vi "Score Display - Show Web Image (LV).vi"(10 "body":string, 11 "Picture in":refnum<vi>) -> ()   [LabVIEW 2013]
uses:
  <vilib>/picture/picture.llb/imagedata.ctl
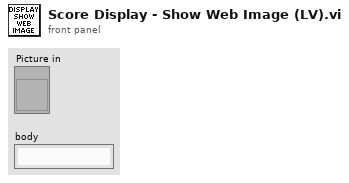
[diagram p1: front panel]
types:
  T1 = typedef "imagedata.ctl" = cluster{"image type":i32, "image depth":i32, "image":u8[], "mask":u8[], "colors":u32[], "Rectangle":cluster{"left":i16, "top":i16, "right":i16, "bottom":i16}}
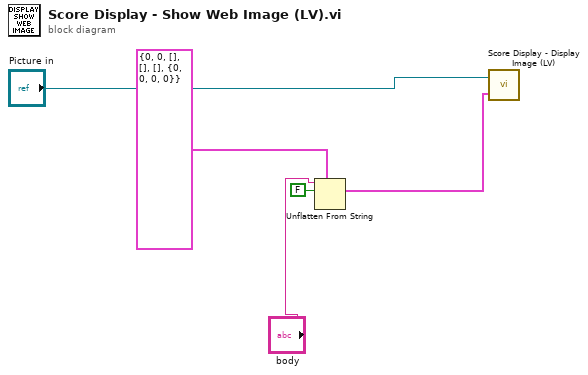
[diagram p0: block diagram]
diagram:
  n1 = Unflatten From String(type=T1 {"image type"=0, "image depth"=0, "image"=[], "mask"=[], "colors"=[], "Rectangle"={"left"=0, "top"=0, "right"=0, "bottom"=0}} ("image data"), binary string="body", data includes array or string size? (T)=FALSE) -> (value=w4:T1)  [unwired: 2 in, 2 out]
  n2 = call "Score Display - Display Image (LV).vi"("image data"=w4, "Picture Reference"="Picture in") -> ()  [unwired: 2 in]
